vi "TicManual.vi"() -> ()   [LabVIEW 2022 SP3]
panel:
  in  "Stop":bool
  out "command string":string
  in  "Frequency(Hz)":dbl=5.204170427930421e-17 step=0.05 format="%.2f"
  # "Set up for Tic running half-steps.\nIf Tic has command timeout set, run this roundy-roundy to keep Tic going"
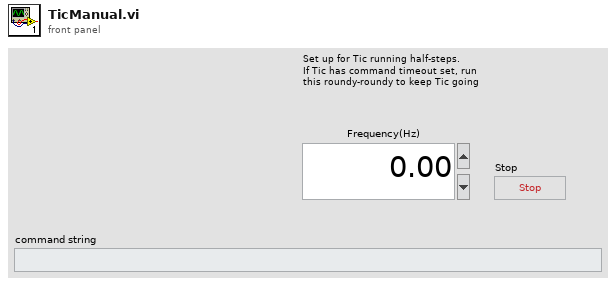
[diagram p1: front panel]
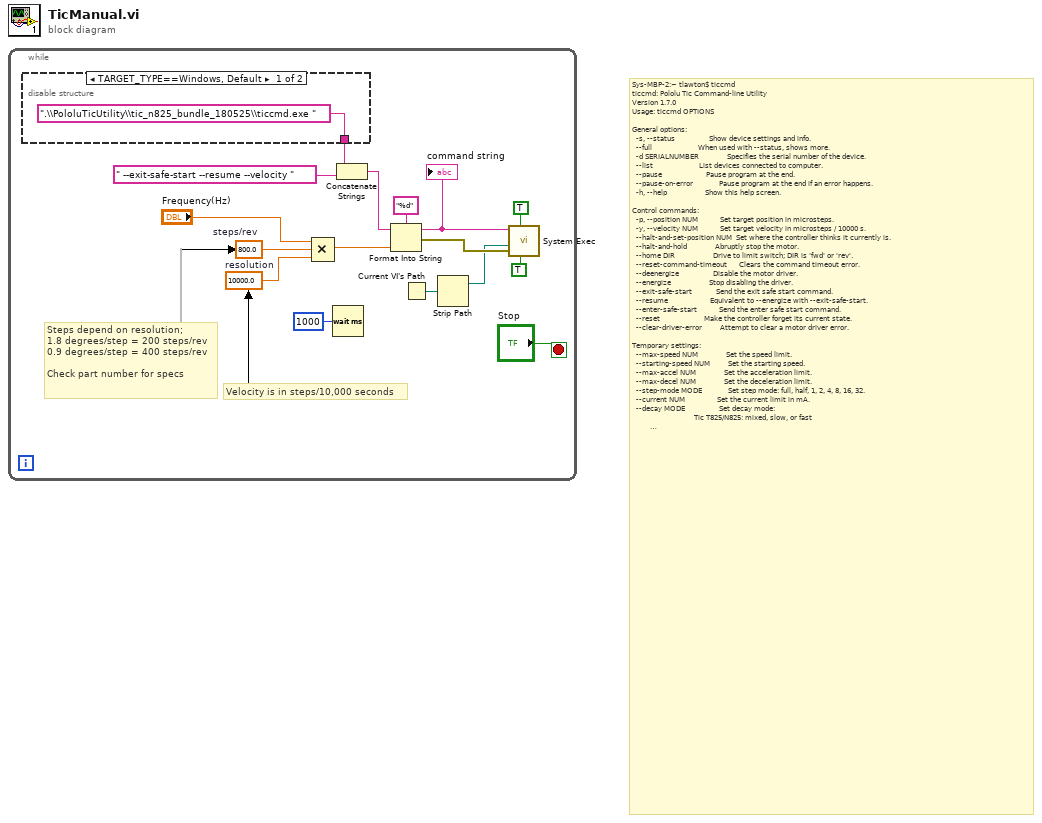
[diagram p0: block diagram]
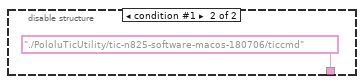
[diagram p2: hidden frame]
diagram:
  # "Sys-MBP-2:~ tlawton$ ticcmd\nticcmd: Pololu Tic Command-line Utility\nVersion 1.7.0\nUsage: ticcmd OPTIONS\n\nGeneral options:\n  -s, --status                 Show device settings and info.\n  --full                       When used with --status, shows more.\n  -d SERIALNUMBER              Specifies the serial number of the device.\n  --list                       List devices connected to computer.\n  --pause                      Pause program at the end.\n  --pause-on-error             Pause program at the end if an error happens.\n  -h, --help                   Show this help screen.\n\nControl commands:\n  -p, --position NUM           Set target position in microsteps.\n  -y, --velocity NUM           Set target velocity in microsteps / 10000 s.\n  --halt-and-set-position NUM  Set where the controller thinks it currently is.\n  --halt-and-hold              Abruptly stop the motor.\n  --home DIR                   Drive to limit switch; DIR is 'fwd' or 'rev'.\n  --reset-command-timeout      Clears the command timeout error.\n  --deenergize                 Disable the motor driver.\n  --energize                   Stop disabling the driver.\n  --exit-safe-start            Send the exit safe start command.\n  --resume                     Equivalent to --energize with --exit-safe-start.\n  --enter-safe-start           Send the enter safe start command.\n  --reset                      Make the controller forget its current state.\n  --clear-driver-error         Attempt to clear a motor driver error.\n\nTemporary settings:\n  --max-speed NUM              Set the speed limit.\n  --starting-speed NUM         Set the starting speed.\n  --max-accel NUM              Set the acceleration limit.\n  --max-decel NUM              Set the deceleration limit.\n  --step-mode MODE             Set step mode: full, half, 1, 2, 4, 8, 16, 32.\n  --current NUM                Set the current limit in mA.\n  --decay MODE                 Set decay mode:\n                               Tic T825/N825: mixed, slow, or fast\n                               T834: slow, mixed25, mixed50, mixed75, or fast\n\nPermanent settings:\n  --restore-defaults           Restore device's factory settings\n  --settings FILE              Load settings file into device.\n  --get-settings FILE          Read device settings and write to file.\n  --fix-settings IN OUT        Read settings from a file and fix them.\n\nFor more help, see: https://www.pololu.com/docs/0J71"
  n1 = while {
    stop <- "Stop" stop-if-true
    w15 = 10000.0  # resolution
    w16 = 800.0  # steps/rev
    # "Velocity is in steps/10,000 seconds"
    # "Steps depend on resolution;\n1.8 degrees/step = 200 steps/rev\n0.9 degrees/step = 400 steps/rev\n\nCheck part number for specs"
    n2 = disable-structure shown="TARGET_TYPE==Windows, Default" {
      disable-tunnel: [".\\PololuTicUtility\\tic_n825_bundle_180525\\ticcmd.exe " ("format string") "./PololuTicUtility/tic-n825-software-macos-180706/ticcmd" ("format string")] -> w6
      frame condition #0 (active) {
      }
      frame condition #1 {
      }
    }
    n3 = Compound Arithmetic op=MULTIPLY("Frequency(Hz)", w16, w15) -> (w14:dbl)
    n4 = Wait (ms)(milliseconds to wait=u32 1000) -> ()  [unwired: 1 out]
    n5 = Concatenate Strings(w6, " --exit-safe-start --resume --velocity ") -> (w5:string)
    n6 = Format Into String(format string="%d", initial string=w5, w14) -> (resulting string=w12:string, error out=w10:errorcluster)  [unwired: 1 in]
    "command string" <- w12
    n7 = Current VI's Path() -> (path=w9:path)
    n8 = Strip Path(path=w9) -> (stripped path=w8:path)  [unwired: 1 out]
    n9 = call <vilib>:"System Exec.vi"("run minimized? (F)"=TRUE, "wait until completion? (T)"=TRUE, "error in (no error)"=w10, "working directory"=w8, "command line"=w12) -> ()  [unwired: 3 in, 4 out]
  }
